vi "solar_excel Export.vi"(4 "Truncate Empty Cells? (F)":bool, 6 "Visible? (F)":bool, 8 "error in (no error)":errorcluster, 10 "TSV Workbook (*.tsv)":path, 11 "Excel Workbook (*.xlsx)":path) -> (0 "error out":errorcluster, 3 "TSV Workbook out":path)   [LabVIEW 2018]
doc: "This exports an Excel Workbook (*.xlsx) into a tab delimited text file (*.tsv). Each Worksheet is separated by section headers (Ex: '[MySheet1]')\n\n[MySheet1]\nA\\tB\\tC\nD\\tE\\tF\n[MySheet2]\n1\\t2\\t3\n4\\t5\\t6"
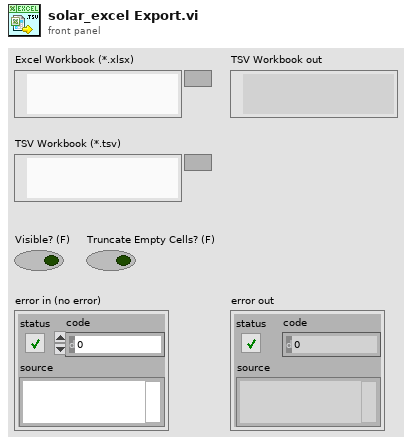
[diagram p1: front panel]
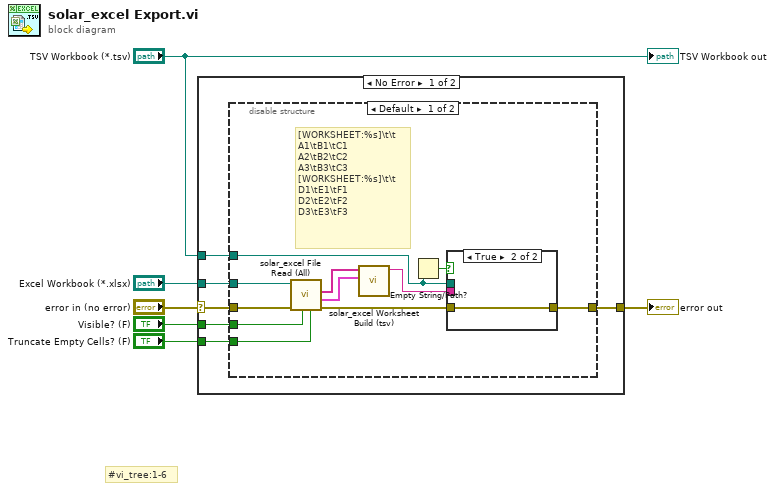
[diagram p0: block diagram]
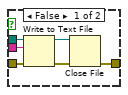
[diagram p2: hidden frame]
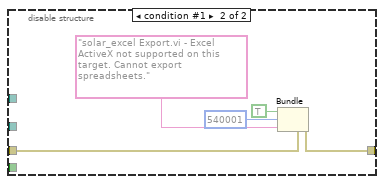
[diagram p3: hidden frame]
diagram:
  # "#vi_tree:1-6"
  n1 = case shown="No Error" "error in (no error)" {
    selector: "error in (no error)" -> [w12 w36]
    tunnel: [w8 w36] -> w5
    tunnel: "Excel Workbook (*.xlsx)" -> [w11 _]
    tunnel: "Visible? (F)" -> [w10 _]
    tunnel: "Truncate Empty Cells? (F)" -> [w9 _]
    tunnel: "TSV Workbook (*.tsv)" -> [w7 _]
    frame No Error {
      n2 = disable-structure shown="Default" {
        disable-tunnel: w12 -> [w23 w33]
        disable-tunnel: w11 -> [w22 _]
        disable-tunnel: w10 -> [w21 _]
        disable-tunnel: w9 -> [w20 _]
        disable-tunnel: [w18 w32] -> w8
        disable-tunnel: w7 -> [w17 _]
        frame condition #0 (active) {
          # "[WORKSHEET:%s]\\t\\t\nA1\\tB1\\tC1\nA2\\tB2\\tC2\nA3\\tB3\\tC3\n[WORKSHEET:%s]\\t\\t\nD1\\tE1\\tF1\nD2\\tE2\\tF2\nD3\\tE3\\tF3"
          n3 = call "solar_excel File Read (All).vi"("Truncate Empty Cells? (F)"=w20, "Visible? (F)"=w21, "error in (no error)"=w23, "Excel Workbook (*.xlsx)"=w22) -> ("error out"=w19:errorcluster, "Worksheets Cells"=w13:cluster{"Cells":string[][]}[], "Worksheets"=w14:string[])  [unwired: 4 in, 1 out]
          n4 = call "solar_excel Worksheet Build (tsv).vi"("Worksheets Cells"=w13, "Worksheets"=w14) -> ("Tab Delimited String"=w15:string)  [unwired: 9 in]
          n5 = Empty String/Path?(string/path=w17) -> (empty?=w16:bool)
          n6 = case shown="True" w16 {
            tunnel: w19 -> [w29 w30]
            tunnel: w17 -> [w28 _]
            tunnel: w15 -> [w27 _]
            tunnel: [w24 w30] -> w18
            frame False {
              n7 = Write to Text File(file (use dialog)=w28, text=w27, error in=w29) -> (refnum out=w25:refnum<file>, error out=w26:errorcluster)  [unwired: 1 in, 1 out]
              n8 = Close File(refnum=w25, error in=w26) -> (error out=w24:errorcluster)  [unwired: 1 out]
            }
            frame True {
            }
          }
        }
        frame condition #1 {
          n9 = Bundle(cluster=w33, "status"=TRUE ("show call chain? (False)"), "code"=540001 ("error code (0)"), "source"="solar_excel Export.vi - Excel ActiveX not supported on this target. Cannot export spreadsheets." ("error message (\"\")")) -> (w32:errorcluster)
        }
      }
    }
    frame Error {
    }
  }
  "error out" <- w5
  "TSV Workbook out" <- "TSV Workbook (*.tsv)"
